vi "Save Buffer to File in the USB.vi"(0 "VISA resource name":refnum<visa-resource-name>, 1 "Add Time Format (T:Enable)":bool, 2 "Full or Partial Data":bool, 5 "Buffer Name (defbuffer1)":string, 7 "File Name":string, 9 "Time format":u16(ring) items=["Format", "Relative", "Raw", "Stamp"], 11 "error in (no error)":errorcluster, 12 "Start":i32, 13 "End":i32) -> (4 "VISA resource name out":refnum<visa-resource-name>, 15 "error out":errorcluster)   [LabVIEW 2009, in "Keithley DMM7510.lvlib"]
doc: "This saves full or partial data from the specified reading buffer to a USB flash drive."
uses:
  Keithley DMM7510.lvlib
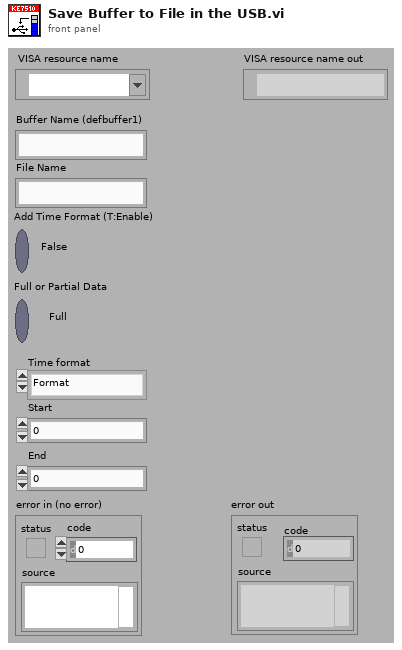
[diagram p1: front panel]
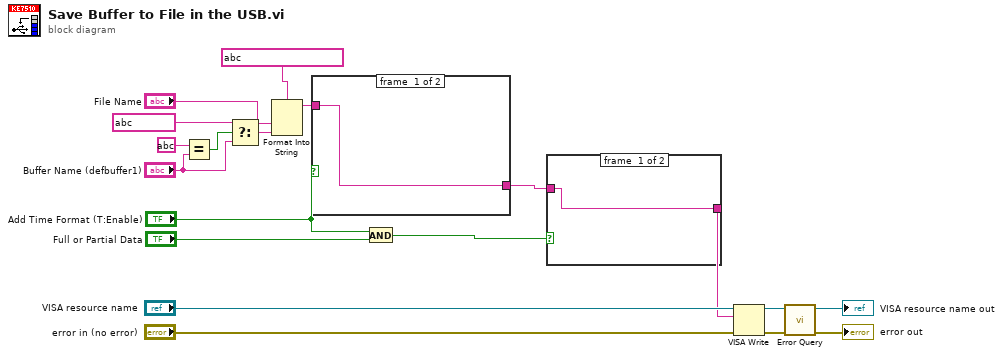
[diagram p0: block diagram]
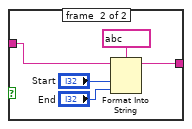
[diagram p2: hidden frame]
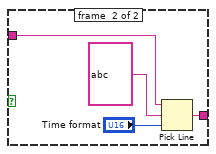
[diagram p3: hidden frame]
diagram:
  n1 = Equal?(x=string ?, y="Buffer Name (defbuffer1)") -> (x = y?=w11:bool)
  n2 = Select(t=string ?, s=w11, f="Buffer Name (defbuffer1)") -> (s? t:f=w7:string)
  n3 = Format Into String(format string=string ? ("Read Measurement"), "File Name", w7) -> (resulting string=w3:string)  [unwired: 2 in, 1 out]
  n4 = case shown="True" "Add Time Format (T:Enable)" {
    tunnel: [w20 w22] -> w2
    tunnel: w3 -> [w20 w21]
    frame #0 {
    }
    frame #1 {
      n5 = Pick Line(string ("")=w21, multi-line string=string ?, line index="Time format") -> (output string=w22:string)
    }
  }
  n6 = And(x="Add Time Format (T:Enable)", y="Full or Partial Data") -> (x .and. y?=w5:bool)
  n7 = case shown="True" w5 {
    tunnel: w2 -> [w25 w27]
    tunnel: [w25 w26] -> w1
    frame #0 {
    }
    frame #1 {
      n8 = Format Into String(format string=string ?, initial string=w27, "Start", "End") -> (resulting string=w26:string)  [unwired: 1 in, 1 out]
    }
  }
  n9 = VISA Write(VISA resource name="VISA resource name", write buffer=w1, error in (no error)="error in (no error)") -> (VISA resource name out=w15:refnum<visa-resource-name>, error out=w14:errorcluster)  [unwired: 1 out]
  n10 = call "Error Query.vi"("error in (no error)"=w14, "VISA resource name"=w15) -> ("error out"=→"error out":errorcluster, "VISA resource name out"=→"VISA resource name out":refnum<visa-resource-name>)  [unwired: 8 out]
